vi "From JSON Tree.vi"(8 "error in (no error)":errorcluster, 10 "JSON in":refnum<class "JSON Null.lvclass">, 11 "id in":refnum<class "id.lvclass">) -> (0 "error out":errorcluster, 3 "id out":refnum<class "id.lvclass">)   [LabVIEW 2015, in "id.lvclass"]
uses:
  id.lvclass
  <vilib>/NI/JSON Support for LabVIEW/JSON Data Classes/JSON Datatype/JSON Null.lvclass
  id.lvclass/id.ctl
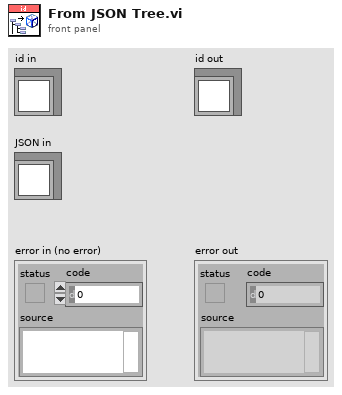
[diagram p1: front panel]
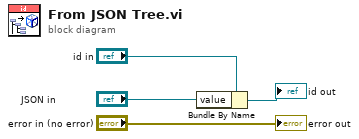
[diagram p0: block diagram]
diagram:
  n1 = Bundle By Name(cluster="id in", "value"="JSON in") -> (→"id out":refnum<class "id.lvclass">)
  "error out" <- "error in (no error)"
